vi "MB test_v3.vi"() -> ()   [LabVIEW 2018, in "MB Relay.lvlib"]
uses:
  MB Relay.lvlib
  type defs/FGV enum.ctl
  <vilib>/NI/Modbus Library/API/Modbus API.lvclass/Modbus API.ctl
  <vilib>/NI/Modbus Library/Transmission Data Unit/Transmission Data Unit.lvclass/Transmission Data Unit.ctl
  <vilib>/NI/Modbus Library/Transmission Data Unit/Write Unit ID.vi
  <vilib>/NI/Modbus Library/API/Read Transmission Data Unit.vi
  <vilib>/NI/Modbus Library/API/Write Transmission Data Unit.vi
  <vilib>/NI/Modbus Library/API/Master/Modbus Master.lvclass
  C:/Program Files (x86)/National Instruments/LabVIEW 2018/vi.lib/NI/Modbus Library/API/Modbus API.lvclass
  <vilib>/ErrorRing/Error Ring.xnode
panel:
  in  "5Venable":bool
  in  "OK Button 3":bool
  in  "OK Button 2":bool
  in  "OK Button":bool
  in  "MB relay01":bool[](array[boolean])=[FALSE, FALSE, FALSE, FALSE, FALSE, FALSE]
  in  "board ID":i32
  in  "Array":bool[](array[boolean])=[FALSE, FALSE, FALSE, FALSE, FALSE, FALSE, FALSE, FALSE, FALSE, FALSE, FALSE, FALSE, FALSE, FALSE, FALSE, FALSE]
  in  "demux1_10(x6)_encode":T1(ring)
  in  "All off":bool
  in  "All On":bool
  out "Holding Regs":u16[](array[numeric]) format="%016b"
  in  "stop":bool
  # "Single Relay (DPDT or SPDT)- Manual Test Mode"
  # "0 -01\n1- 11\n2- 12\n3-13\n4-14\n5 - 21\n6-22\n7-23\n8-24\n9-30\n10-31"
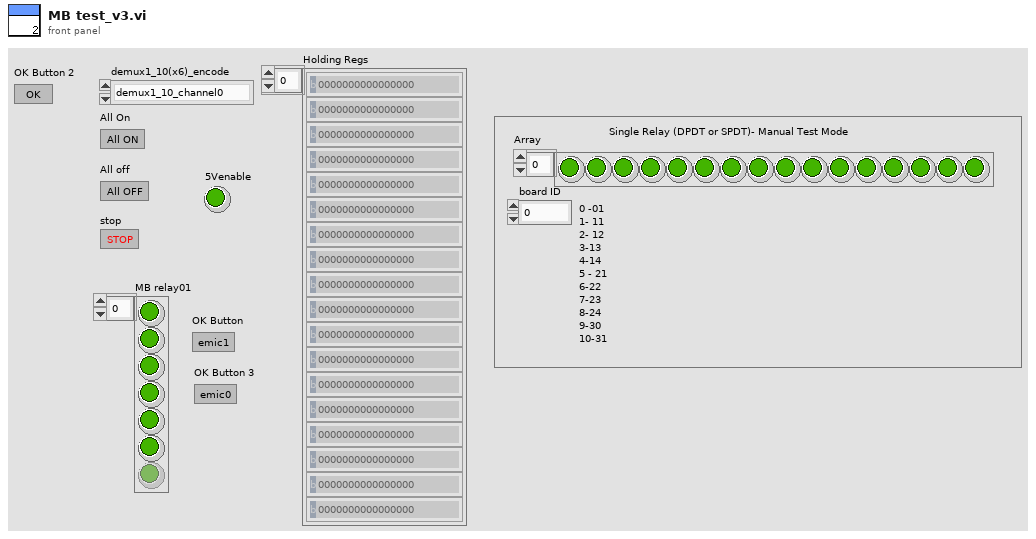
[diagram p1: front panel]
types:
  T1 = enum16{"demux1_10_channel0", "demux1_10_channel1", "demux1_10_channel2", "demux1_10_channel3", "demux1_10_channel4", "demux1_10_channel5", "demux1_10_channel6", "demux1_10_channel7", "demux1_10_channel8", "demux1_10_channel9", "demux1_10_channel10"}
  T2 = typedef "MB Relay.lvlib/FGV enum.ctl" = enum16{"Write", "Read", "All OFF", "All ON"}
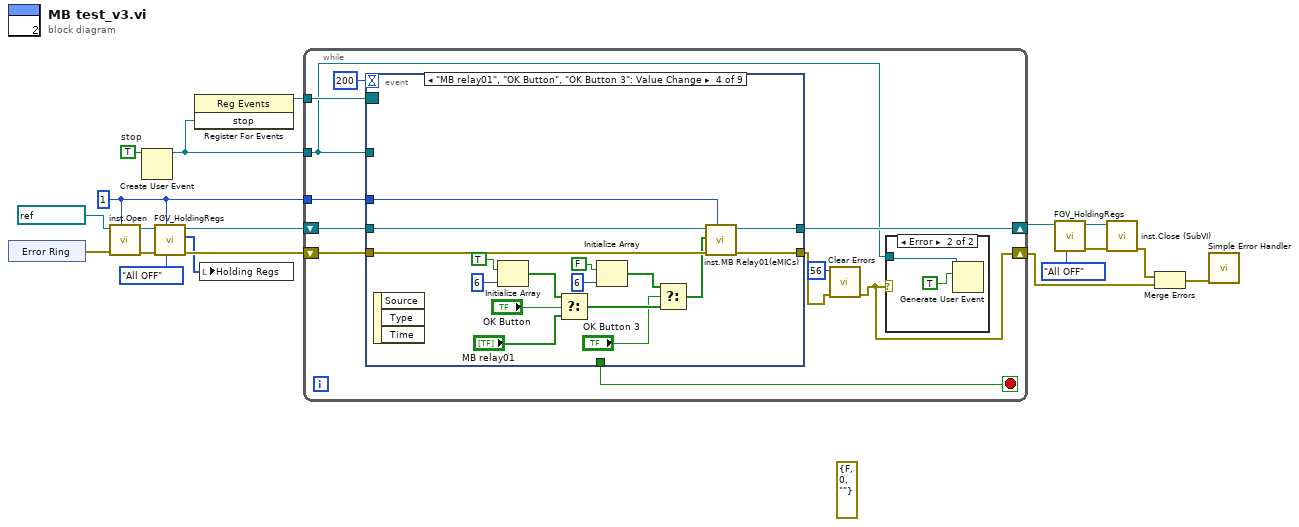
[diagram p0: block diagram]
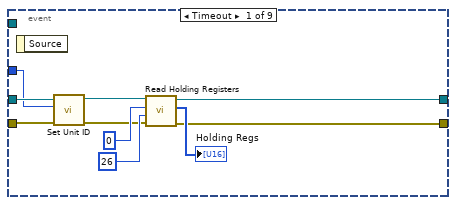
[diagram p3: hidden frame]
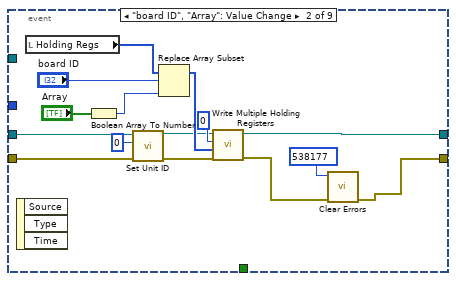
[diagram p4: hidden frame]
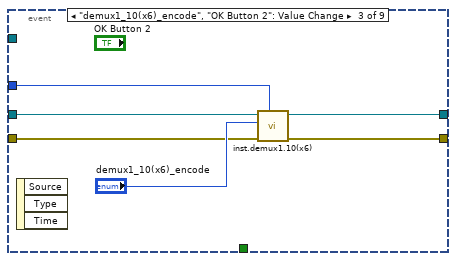
[diagram p5: hidden frame]
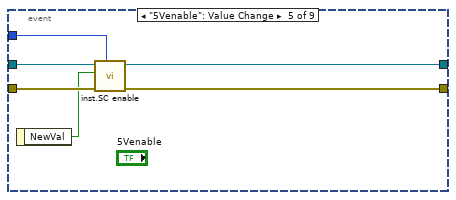
[diagram p6: hidden frame]
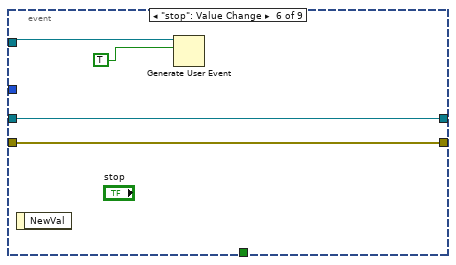
[diagram p7: hidden frame]
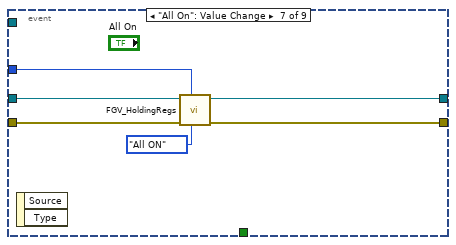
[diagram p8: hidden frame]
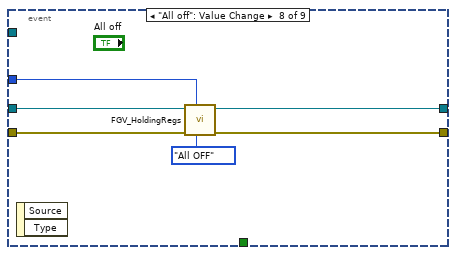
[diagram p9: hidden frame]
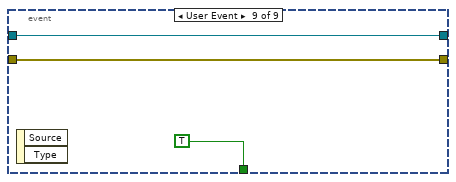
[diagram p10: hidden frame]
diagram:
  (unwired) errorcluster {"status"=FALSE, "code"=0, "source"=""} ("error IO")
  w18 = TRUE  # stop
  w7 = u8 1 ("unit ID in")
  n1 = xnode "Error Ring"() -> ("error out"=w19:errorcluster)
  n2 = call "inst.Open.vi"("unit ID in"=w7, "error in (no error)"=w19, "VISA resource name"=refnum<visa-resource-name> "COM16") -> ("error out"=w12:errorcluster, "Modbus Master out"=w11:refnum<class "Modbus Master.lvclass">)  [unwired: 7 in]
  n3 = Create User Event(user event datatype=w18) -> (user event=w16:refnum<user-event>)  [unwired: 1 in, 1 out]
  n4 = call "FGV_HoldingRegs.vi"("FGV_enum"=FGV_enum."All OFF", "unit ID"=w7, "error in (no error)"=w12, "Modbus master in"=w11) -> ("error out"=w9:errorcluster, "HoldingRegs"=w8:u16[], "Modbus master out"=w10:refnum<class "Modbus Master.lvclass">)  [unwired: 5 in]
  n5 = register-events(w16) -> (reference out=w17:refnum<event-registration>)  [unwired: 2 in, 1 out]
  n6 = local write "Holding Regs"(w8) -> ()
  n7 = while {
    shift-right: [w26] -> w3
    shift-left: w10 -> [w29]
    tunnel: w17 -> [w25]
    tunnel: w16 -> [w24]
    tunnel: w7 -> [w23]
    shift-right: [w20] -> w6
    shift-left: w9 -> [w28]
    stop <- w30 stop-if-true
    n8 = event shown="[3] \"MB relay01\", \"OK Button\", \"OK Button 3\": Value Change" {
      selector: w25 -> [_ _ _ _ _ _ _ _ _]
      dyn-events: _ -> [_ _ _ _ _ _ _ _ _]
      timeout: 200 -> [_ _ _ _ _ _ _ _ _]
      tunnel: [_ _ _ _ _ _ _ _ TRUE] -> w30
      tunnel: w29 -> [w36 w50 w62 w79 w85 w87 w95 w101 w103]
      tunnel: w28 -> [w37 w49 w60 w78 w84 w86 w94 w98 w102]
      tunnel: [w42 w53 w58 w77 w82 w87 w91 w99 w103] -> w26
      tunnel: [w38 w44 w59 w76 w81 w86 w92 w97 w102] -> w21
      tunnel: w24 -> [_ _ _ _ _ w89 _ _ _]
      tunnel: w23 -> [w35 _ w61 w75 w83 _ w90 w100 _]
      event Timeout {
        n9 = event-data() -> ()  [unwired: 1 in, 1 out]
        n10 = call <vilib>:"Set Unit ID.vi"("error in"=w37, "unit ID"=w35, "Modbus master in"=w36) -> ("error out"=w33:errorcluster, "Modbus master out"=w34:refnum<class "Modbus Master.lvclass">)  [unwired: 7 in]
        n11 = call-dynamic "Read Holding Registers.vi"("error in"=w33, "number of inputs"=u16 26, "starting address"=u16 0, "Modbus master in"=w34) -> ("error out"=w38:errorcluster, "register values"=→"Holding Regs":u16[], "Modbus master out"=w42:refnum<class "Modbus Master.lvclass">)  [unwired: 5 in]
      }
      event "board ID", "Array": Value Change {
        n12 = event-data() -> ()  [unwired: 1 in, 3 out]
        n13 = local read "Holding Regs"() -> (w56:u16[])
        n14 = Boolean Array To Number(Boolean array="Array") -> (number=w54:u16)
        n15 = call <vilib>:"Set Unit ID.vi"("error in"=w49, "unit ID"=u8 0, "Modbus master in"=w50) -> ("error out"=w48:errorcluster, "Modbus master out"=w47:refnum<class "Modbus Master.lvclass">)  [unwired: 7 in]
        n16 = Replace Array Subset(array=w56, new element=w54, index="board ID") -> (w52:u16[])
        n17 = call-dynamic "Write Multiple Holding Registers.vi"("error in"=w48, "registers to write"=w52, "starting address"=u16 0, "Modbus master in"=w47) -> ("error out"=w45:errorcluster, "Modbus master out"=w53:refnum<class "Modbus Master.lvclass">)  [unwired: 6 in]
        n18 = call <vilib>:"Clear Errors.vi"("error in (no error)"=w45, "specific error code to clear (0: all)"=538177) -> ("error out"=w44:errorcluster)  [unwired: 4 in, 1 out]
      }
      event "demux1_10(x6)_encode", "OK Button 2": Value Change {
        n19 = event-data() -> ()  [unwired: 1 in, 3 out]
        n20 = call "inst.demux1.10(x6).vi"("unit ID"=w61, "error in (no error)"=w60, "demux1_10(x6)_encode"="demux1_10(x6)_encode", "Modbus Master in"=w62) -> ("error out"=w59:errorcluster, "Modbus Master out"=w58:refnum<class "Modbus Master.lvclass">)  [unwired: 6 in]
      }
      event "MB relay01", "OK Button", "OK Button 3": Value Change {
        n21 = event-data() -> ()  [unwired: 1 in, 3 out]
        n22 = Initialize Array(TRUE, 6 ("dimension size")) -> (w70:bool[])
        n23 = Select(t=w70, s="OK Button", f="MB relay01") -> (s? t:f=w67:bool[])
        n24 = Initialize Array(FALSE, 6 ("dimension size")) -> (w66:bool[])
        n25 = Select(t=w66, s="OK Button 3", f=w67) -> (s? t:f=w64:bool[])
        n26 = call "inst.MB Relay01(eMICs).vi"("unit ID"=w75, "error in (no error)"=w78, "MB relay01"=w64, "Modbus Master in"=w79) -> ("error out"=w76:errorcluster, "Modbus Master out"=w77:refnum<class "Modbus Master.lvclass">)  [unwired: 6 in]
      }
      event "5Venable": Value Change {
        n27 = event-data() -> ("NewVal"=w80:bool)  [unwired: 1 in]
        n28 = call "inst.SC enable.vi"("unit ID"=w83, "error in (no error)"=w84, "5V enable"=w80, "Modbus Master in"=w85) -> ("error out"=w81:errorcluster, "Modbus Master out"=w82:refnum<class "Modbus Master.lvclass">)  [unwired: 6 in]
      }
      event "stop": Value Change {
        n29 = event-data() -> ()  [unwired: 1 in, 1 out]
        n30 = Generate User Event(user event=w89, event data cluster=TRUE) -> ()  [unwired: 2 in, 2 out]
      }
      event "All On": Value Change {
        n31 = event-data() -> ()  [unwired: 1 in, 2 out]
        n32 = call "FGV_HoldingRegs.vi"("FGV_enum"=FGV_enum."All ON", "unit ID"=w90, "error in (no error)"=w94, "Modbus master in"=w95) -> ("error out"=w92:errorcluster, "Modbus master out"=w91:refnum<class "Modbus Master.lvclass">)  [unwired: 5 in, 1 out]
      }
      event "All off": Value Change {
        n33 = event-data() -> ()  [unwired: 1 in, 2 out]
        n34 = call "FGV_HoldingRegs.vi"("FGV_enum"=FGV_enum."All OFF", "unit ID"=w100, "error in (no error)"=w98, "Modbus master in"=w101) -> ("error out"=w97:errorcluster, "Modbus master out"=w99:refnum<class "Modbus Master.lvclass">)  [unwired: 5 in, 1 out]
      }
      event User Event {
        n35 = event-data() -> ()  [unwired: 1 in, 2 out]
      }
    }
    n36 = call <vilib>:"Clear Errors.vi"("error in (no error)"=w21, "specific error code to clear (0: all)"=56) -> ("error out"=w20:errorcluster)  [unwired: 4 in, 1 out]
    n37 = case shown="Error" w20 {
      tunnel: w24 -> [_ w32]
      frame No Error {
      }
      frame Error {
        n38 = Generate User Event(user event=w32, event data cluster=TRUE) -> ()  [unwired: 2 in, 2 out]
      }
    }
  }
  n39 = call "FGV_HoldingRegs.vi"("FGV_enum"=FGV_enum."All OFF", "Modbus master in"=w3) -> ("error out"=w1:errorcluster, "Modbus master out"=w2:refnum<class "Modbus Master.lvclass">)  [unwired: 7 in, 1 out]
  n40 = call "inst.Close (SubVI).vi"("error in (no error)"=w1, "Modbus Master in"=w2) -> ("error out"=w15:errorcluster)  [unwired: 9 in]
  n41 = Merge Errors(w15, w6) -> (w14:errorcluster)
  n42 = call <vilib>:"Simple Error Handler.vi"("error in (no error)"=w14) -> ()  [unwired: 4 in, 5 out]
